vi "Sort Relays.vi"(11 "Relays":T1[](array[typedef])) -> (3 "Sorted Relays":T1[](array[typedef]))   [LabVIEW 2013, in "MUX Custom Device.lvlib"]
uses:
  MUX Custom Device.lvlib
  Relay Status.ctl
  Relay Data.ctl
  Switch.ctl
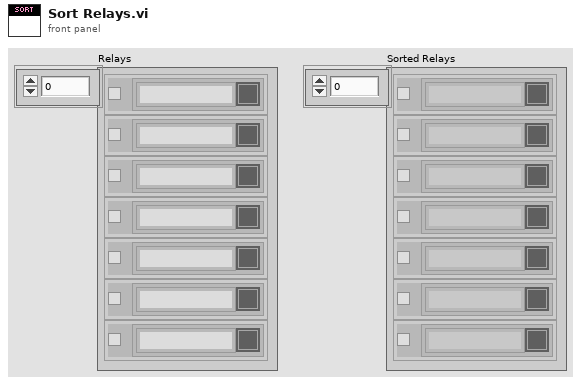
[diagram p1: front panel]
types:
  T1 = typedef "MUX Custom Device.lvlib/Relay Status.ctl" = cluster{"Present":bool, "Relay Data":T2}
  T2 = typedef "MUX Custom Device.lvlib/Relay Data.ctl" = cluster{"Relay Name":string, "State":T3}
  T3 = typedef "MUX Custom Device.lvlib/Switch.ctl" = bool
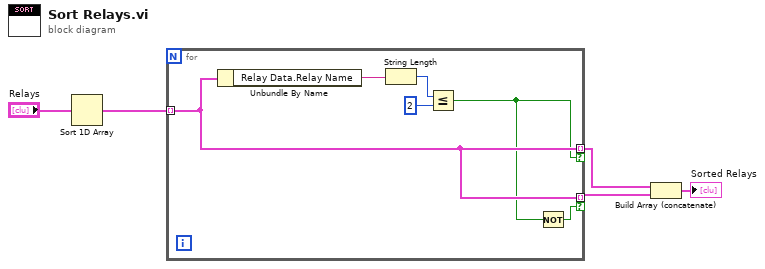
[diagram p0: block diagram]
diagram:
  n1 = Sort 1D Array(array="Relays") -> (sorted array=w4:T1[])
  n2 = for {
    tunnel: w4 -> [w8] mode=indexing
    tunnel: [w8] -> w3 mode=indexing if=w7
    tunnel: [w8] -> w2 mode=indexing if=w6
    n3 = Unbundle By Name(w8) -> ("Relay Data.Relay Name"=w11:string)
    n4 = String Length(string=w11) -> (length=w10:i32)
    n5 = Less Or Equal?(x=w10, y=2) -> (x <= y?=w7:bool)
    n6 = Not(x=w7) -> (.not. x?=w6:bool)
  }
  n7 = Build Array (concatenate)(w3, w2) -> (→"Sorted Relays":T1[])
